vi "LVClass_CameraSet Get Parameter Bool Value.vi"(0 "CameraSet.lvclass":refnum<class "CameraSet.lvclass">, 5 "parameter_name":string, 11 "error in (no error)":errorcluster) -> (4 "CameraSet.lvclass":refnum<class "CameraSet.lvclass">, 6 "Value":bool, 15 "error out":errorcluster)   [LabVIEW 2020, in "CameraSet.lvclass"]
doc: "Camera parameter value getter for parameter of type boolean.\n\n<B>camera_setIn</B> : CameraSet object.\n<B>camera_setOut</B> : CameraSet object.\n<B>parameter_name</B> : Parameter name.\n<B>value</B> : Parameter value."
uses:
  CameraSet.lvclass
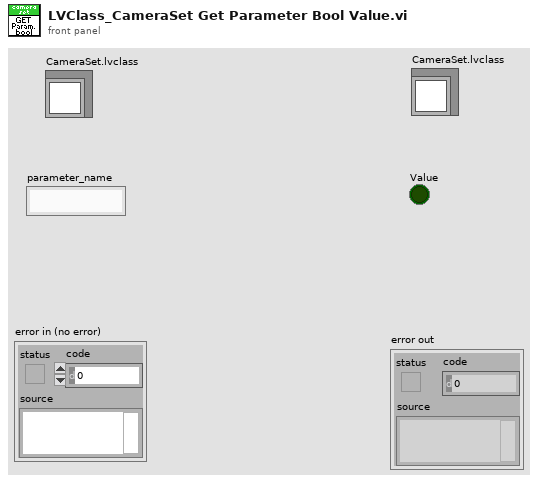
[diagram p1: front panel]
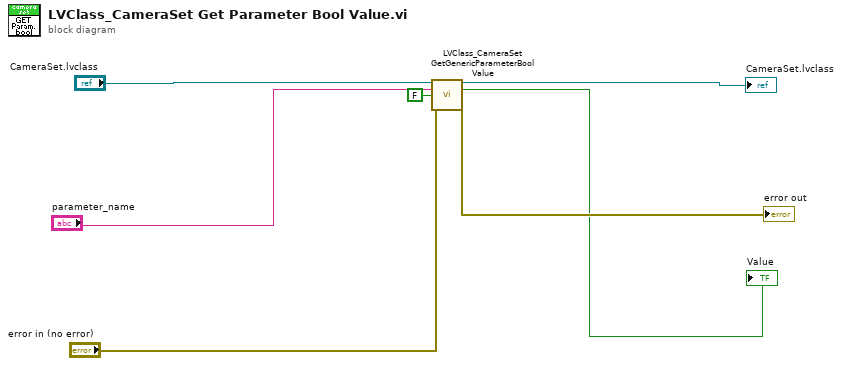
[diagram p0: block diagram]
diagram:
  n1 = call "LVClass_CameraSet GetGenericParameterBoolValue.vi"("CameraSet.lvclass"="CameraSet.lvclass", "parameter_name"="parameter_name", "DefaultFactorySet"=FALSE, "error in (no error)"="error in (no error)") -> ("CameraSet.lvclass"=→"CameraSet.lvclass":refnum<class "CameraSet.lvclass">, "Value"=→"Value":bool, "error out"=→"error out":errorcluster)  [unwired: 9 in]
